vi "write_return_distance.vi"(8 "error in (no error)":errorcluster, 10 "return_distance":bool=TRUE, 11 "KNeighbors in":refnum<class "KNeighbors.lvclass">) -> (0 "error out":errorcluster, 3 "KNeighbors out":refnum<class "KNeighbors.lvclass">)   [LabVIEW 2020, in "KNeighbors.lvclass"]
uses:
  KNeighbors.lvclass
  KNeighbors.lvclass/KNeighbors.ctl
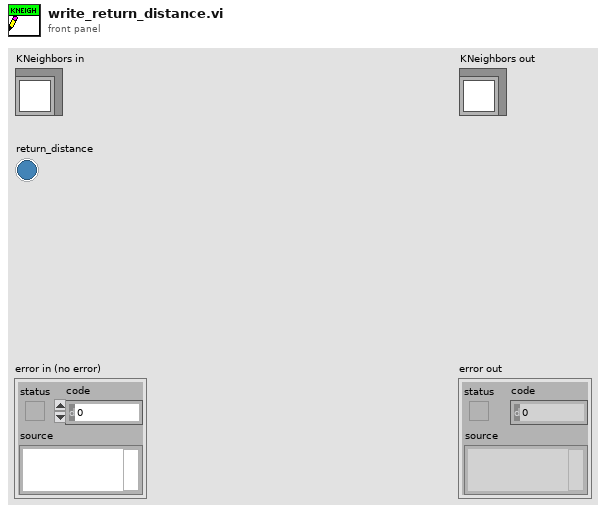
[diagram p1: front panel]
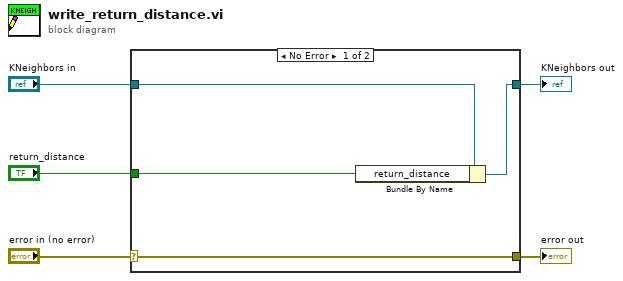
[diagram p0: block diagram]
diagram:
  n1 = case shown="No Error" "error in (no error)" {
    selector: "error in (no error)" -> [w9 w10]
    tunnel: [w9 w10] -> w4
    tunnel: [w7 w11] -> w2
    tunnel: "KNeighbors in" -> [w8 w11]
    tunnel: "return_distance" -> [w6 _]
    frame No Error {
      n2 = Bundle By Name(cluster=w8, "return_distance"=w6) -> (w7:refnum<class "KNeighbors.lvclass">)
    }
    frame Error {
    }
  }
  "error out" <- w4
  "KNeighbors out" <- w2
